vi "Play Preview.vi"() -> ()   [LabVIEW 2013]
doc: "This example VI demonstrates how to acquire and display the preview image from a Phantom Camera using the Vision Research Phantom Series LabVIEW Driver. Also demonstrated is the creation of an image histogram."
uses:
  _Type Defs/PhInt Color.ctl
  _Type Defs/PhInt PhProcessImage Selectors.ctl
  _Type Defs/PhInt REDUCE16TO8PARAMS.ctl
  _Type Defs/PHCon IMRANGE.ctl
  _Type Defs/PhFile InfName.ctl
  _Type Defs/PhFile PRANGE.ctl
  VRI.lvlib
panel:
  in  "REDUCE16TO8PARAMS":T1={"fGain16_8"=1.0}
  in  "procID":T2=1 items=["IMG_PROC_REDUCE16TO8"=1]
  out "Preview":picture
  in  "stop":bool
  in  "Color":T3
  out "pAvgB":u32
  out "pAvgG":u32
  out "pAvgR":u32
  out "Histogram":u32[](graph)
  out "Error Out":errorcluster
  in  "Camera Number":u32
  in  "error in (no error)":errorcluster
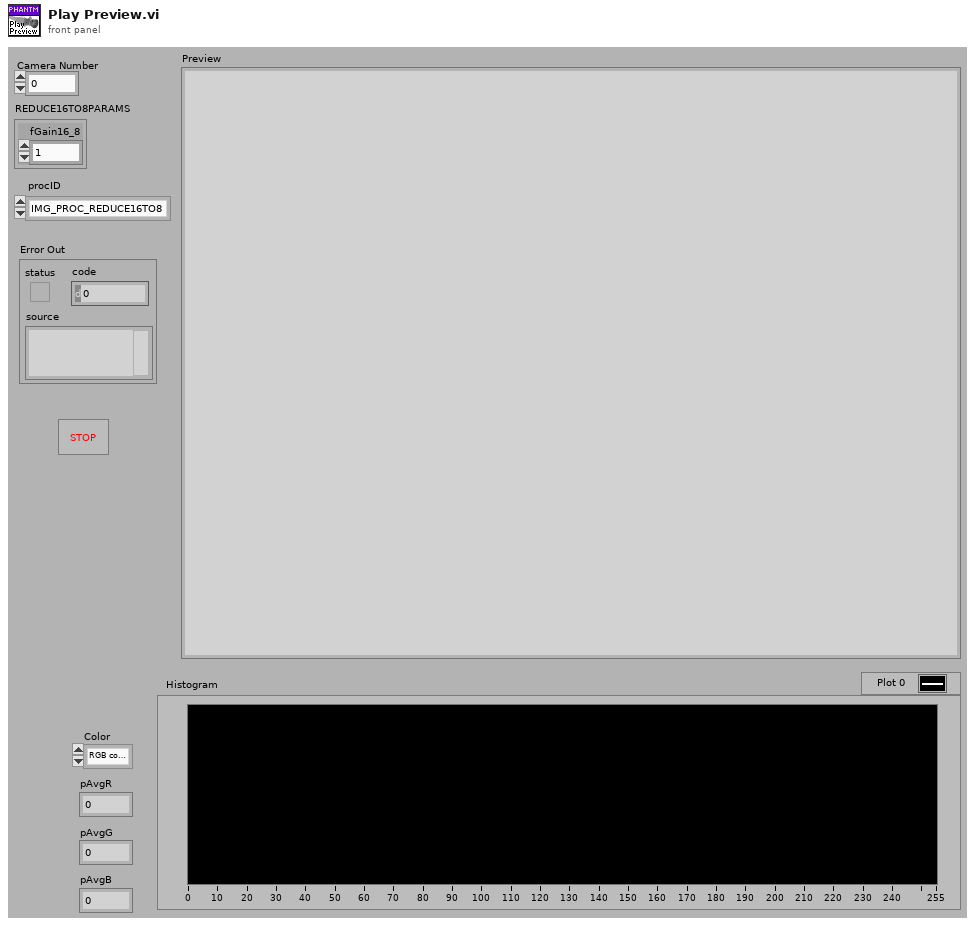
[diagram p1: front panel]
types:
  T1 = typedef "VRI.lvlib/PhInt REDUCE16TO8PARAMS.ctl" = cluster{"fGain16_8":dbl}
  T2 = typedef "VRI.lvlib/PhInt PhProcessImage Selectors.ctl" = u16
  T3 = typedef "VRI.lvlib/PhInt Color.ctl" = enum32{"RGB converted to gray", "RED", "GREEN", "BLUE"}
  T4 = typedef "VRI.lvlib/PhFile PRANGE.ctl" = cluster{"First":u32, "Count":u32}
  T5 = typedef "VRI.lvlib/PhFile InfName.ctl" = u32
  T6 = typedef "VRI.lvlib/PHCon IMRANGE.ctl" = cluster{"First":i32, "Cnt":u32}
  T7 = typedef "VRI.lvlib/PhInt IH.ctl" = cluster{"biSize":u32, "biWidth":i32, "biHeight":i32, "biPlanes":u16, "biBitCount":u16, "biCompresssion":u32, "biSizeImage":u32, "biXPelsPerMeter":i32, "biYPelsPerMeter":i32, "biClrUsed":u32, "biClrImportant":u32, "BlackLevel":i32, "WhiteLevel":i32}
  T8 = typedef "VRI.lvlib/BITMAPINFOHEADER.ctl" = cluster{"biSize":u32, "biWidth":i32, "biHeight":i32, "biPlanes":u16, "biBitCount":u16, "biCompression":u32, "biSizeImage":u32, "biXPelsPerMeter":i32, "biYPelsPerMeter":i32, "biClrUsed":u32, "biClrImportant":u32}
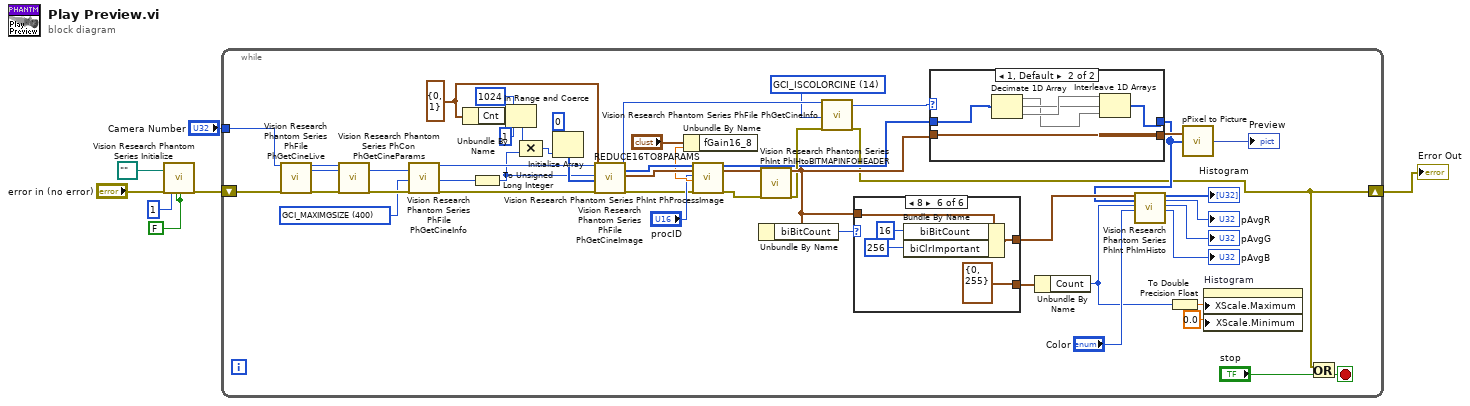
[diagram p0: block diagram]
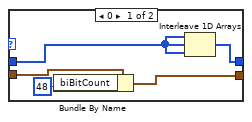
[diagram p2: hidden frame]
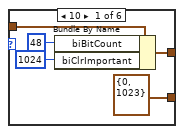
[diagram p3: hidden frame]
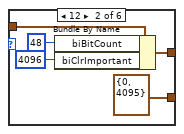
[diagram p4: hidden frame]
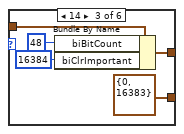
[diagram p5: hidden frame]
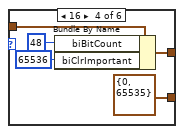
[diagram p6: hidden frame]
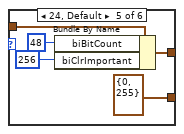
[diagram p7: hidden frame]
diagram:
  w4 = FALSE ("ID Query (T: Check)")
  n1 = call "Vision Research Phantom Series Initialize.vi"("Storage Path (\"\")"=path "" ("Storage Path (\"\")"), "error in (no error)"="error in (no error)", "CallID"=u32 1, "ID Query (T: Check)"=w4, "Reset (F: Don't Reset)"=w4) -> ("Error Out"=w2:errorcluster)  [unwired: 14 out]
  n2 = while {
    tunnel: "Camera Number" -> [w25]
    shift-right: [w8] -> w1
    shift-left: w2 -> [w21]
    stop <- w9 stop-if-true
    w10 = T5 14 items=["GCI_CFA"=0, "GCI_FRAMERATE"=1, "GCI_EXPOSURE"=2, "GCI_AUTOEXPOSURE"=3, "GCI_REALBPP"=4, "GCI_CAMERASERIAL"=5, "GCI_HEADSERIAL0"=6, "GCI_HEADSERIAL1"=7, "GCI_HEADSERIAL2"=8, "GCI_HEADSERIAL3"=9, "GCI_TRIGTIMESEC"=10, "GCI_TRIGTIMEFR"=11, "GCI_ISFILECINE"=12, "GCI_IS16BPPCINE"=13, "GCI_ISCOLORCINE"=14, "GCI_ISMULTIHEADCINE"=15, "GCI_EXPOSURENS"=16, "GCI_EDREXPOSURENS"=17, "GCI_FRAMEDELAYNS"=19, "GCI_FROMFILETYPE"=20, "GCI_COMPRESSION"=21, "GCI_CAMERAVERSION"=22, "GCI_ROTATE"=23, "GCI_IMWIDTH"=24, "GCI_IMHEIGHT"=25, "GCI_IMWIDTHACQ"=26, "GCI_IMHEIGHTACQ"=27, "GCI_POSTTRIGGER"=28, "GCI_IMAGECOUNT"=29, "GCI_TOTALIMAGECOUNT"=30, "GCI_TRIGFRAME"=31, "GCI_AUTOEXPLEVEL"=32, "GCI_AUTOEXPTOP"=33, "GCI_AUTOEXPLEFT"=34, "GCI_AUTOEXPBOTTOM"=35, "GCI_AUTOEXPRIGHT"=36, "GCI_RECORDINGTIMEZONE"=37, "GCI_FIRSTIMAGENO"=38, "GCI_FIRSTMOVIEIMAGE"=39, "GCI_CINENAME"=40, "GCI_FRPSTEPS"=100, "GCI_FRP1X"=101, "GCI_FRP1Y"=102, "GCI_FRP2X"=103, "GCI_FRP2Y"=104, "GCI_FRP3X"=105, "GCI_FRP3Y"=106, "GCI_FRP4X"=107, "GCI_FRP4Y"=108, "GCI_WRITEERR"=109, "GCI_LENSDESCRIPTION"=110, "GCI_LENSAPERATURE"=111, "GCI_LENSFOCALLENGTH"=112, "GCI_WB"=200, "GCI_WBVIEW"=201, "GCI_BRIGHT"=202, "GCI_CONTRAST"=203, "GCI_GAMMA"=204, "GCI_GAMMAR"=223, "GCI_GAMMAB"=224, "GCI_SATURATION"=205, "GCI_HUE"=206, "GCI_FLIPH"=207, "GCI_FLIPV"=208, "GCI_FILTERCODE"=209, "GCI_IMFILTER"=210, "GCI_INTALGO"=211, "GCI_PEDESTALR"=212, "GCI_PEDESTALG"=213, "GCI_PEDESTALB"=214, "GCI_FLARE"=225, "GCI_CHROMA"=226, "GCI_TONE"=227, "GCI_ENABLEMATRICES"=228, "GCI_USERMATRIX"=229, "GCI_RESAMPLEACTIVE"=215, "GCI_RESAMPLEWIDTH"=216, "GCI_RESAMPLEHEIGHT"=217, "GCI_CROPACTIVE"=218, "GCI_CROPRECTANGLE"=219, "GCI_OFFSET16_8"=220, "GCI_GAIN16_8"=221, "GCI_DEMOSAICINGFUNCPTR"=222, "GCI_VFLIPVIEWACTIVE"=300, "GCI_MAXIMGSIZE"=400, "GCI_FRPIMGNOARRAY"=450, "GCI_FRPRATEARRAY"=451, "GCI_FRPSHAPEARRAY"=452, "GCI_TRIGTC"=470, "GCI_TRIGTCU"=471, "GCI_PBRATE"=472, "GCI_TCRATE"=473, "GCI_SAVERANGE"=500, "GCI_SAVEFILENAME"=501, "GCI_SAVEFILETYPE"=502, "GCI_SAVE16BIT"=503, "GCI_SAVEPACKED"=504, "GCI_SAVEXML"=505, "GCI_SAVESTAMPTIME"=506, "GCI_SAVEAVIFRAMERATE"=520, "GCI_SAVEAVICOMPRESSORLIST"=521, "GCI_SAVEAVICOMPRESSORINDEX"=522, "GCI_SAVEDPXLSB"=530, "GCI_SAVEDPXTO10BPS"=531, "GCI_SAVEDPXDATAPACKING"=532, "GCI_SAVEDPX10BITLOG"=533, "GCI_SAVEDPXEXPORTLOGLUT"=534, "GCI_SAVEDPX10BITLOGREFWHITE"=535, "GCI_SAVEDPX10BITLOGREFBLACK"=536, "GCI_SAVEDPX10BITLOGGAMMA"=537, "GCI_SAVEDPX10BITLOGFILMGAMMA"=538, "GCI_SAVEQTPLAYBACKRATE"=550, "GCI_SAVECCIQUALITY"=560, "GCI_UNCALIBRATEDIMAGE"=600, "GCI_NOPROCESSING"=601, "GCI_BADPIXELREPAIR"=602] ("InfName")
    w22 = T5 400 items=["GCI_CFA"=0, "GCI_FRAMERATE"=1, "GCI_EXPOSURE"=2, "GCI_AUTOEXPOSURE"=3, "GCI_REALBPP"=4, "GCI_CAMERASERIAL"=5, "GCI_HEADSERIAL0"=6, "GCI_HEADSERIAL1"=7, "GCI_HEADSERIAL2"=8, "GCI_HEADSERIAL3"=9, "GCI_TRIGTIMESEC"=10, "GCI_TRIGTIMEFR"=11, "GCI_ISFILECINE"=12, "GCI_IS16BPPCINE"=13, "GCI_ISCOLORCINE"=14, "GCI_ISMULTIHEADCINE"=15, "GCI_EXPOSURENS"=16, "GCI_EDREXPOSURENS"=17, "GCI_FRAMEDELAYNS"=19, "GCI_FROMFILETYPE"=20, "GCI_COMPRESSION"=21, "GCI_CAMERAVERSION"=22, "GCI_ROTATE"=23, "GCI_IMWIDTH"=24, "GCI_IMHEIGHT"=25, "GCI_IMWIDTHACQ"=26, "GCI_IMHEIGHTACQ"=27, "GCI_POSTTRIGGER"=28, "GCI_IMAGECOUNT"=29, "GCI_TOTALIMAGECOUNT"=30, "GCI_TRIGFRAME"=31, "GCI_AUTOEXPLEVEL"=32, "GCI_AUTOEXPTOP"=33, "GCI_AUTOEXPLEFT"=34, "GCI_AUTOEXPBOTTOM"=35, "GCI_AUTOEXPRIGHT"=36, "GCI_RECORDINGTIMEZONE"=37, "GCI_FIRSTIMAGENO"=38, "GCI_FIRSTMOVIEIMAGE"=39, "GCI_CINENAME"=40, "GCI_FRPSTEPS"=100, "GCI_FRP1X"=101, "GCI_FRP1Y"=102, "GCI_FRP2X"=103, "GCI_FRP2Y"=104, "GCI_FRP3X"=105, "GCI_FRP3Y"=106, "GCI_FRP4X"=107, "GCI_FRP4Y"=108, "GCI_WRITEERR"=109, "GCI_LENSDESCRIPTION"=110, "GCI_LENSAPERATURE"=111, "GCI_LENSFOCALLENGTH"=112, "GCI_WB"=200, "GCI_WBVIEW"=201, "GCI_BRIGHT"=202, "GCI_CONTRAST"=203, "GCI_GAMMA"=204, "GCI_GAMMAR"=223, "GCI_GAMMAB"=224, "GCI_SATURATION"=205, "GCI_HUE"=206, "GCI_FLIPH"=207, "GCI_FLIPV"=208, "GCI_FILTERCODE"=209, "GCI_IMFILTER"=210, "GCI_INTALGO"=211, "GCI_PEDESTALR"=212, "GCI_PEDESTALG"=213, "GCI_PEDESTALB"=214, "GCI_FLARE"=225, "GCI_CHROMA"=226, "GCI_TONE"=227, "GCI_ENABLEMATRICES"=228, "GCI_USERMATRIX"=229, "GCI_RESAMPLEACTIVE"=215, "GCI_RESAMPLEWIDTH"=216, "GCI_RESAMPLEHEIGHT"=217, "GCI_CROPACTIVE"=218, "GCI_CROPRECTANGLE"=219, "GCI_OFFSET16_8"=220, "GCI_GAIN16_8"=221, "GCI_DEMOSAICINGFUNCPTR"=222, "GCI_VFLIPVIEWACTIVE"=300, "GCI_MAXIMGSIZE"=400, "GCI_FRPIMGNOARRAY"=450, "GCI_FRPRATEARRAY"=451, "GCI_FRPSHAPEARRAY"=452, "GCI_TRIGTC"=470, "GCI_TRIGTCU"=471, "GCI_PBRATE"=472, "GCI_TCRATE"=473, "GCI_SAVERANGE"=500, "GCI_SAVEFILENAME"=501, "GCI_SAVEFILETYPE"=502, "GCI_SAVE16BIT"=503, "GCI_SAVEPACKED"=504, "GCI_SAVEXML"=505, "GCI_SAVESTAMPTIME"=506, "GCI_SAVEAVIFRAMERATE"=520, "GCI_SAVEAVICOMPRESSORLIST"=521, "GCI_SAVEAVICOMPRESSORINDEX"=522, "GCI_SAVEDPXLSB"=530, "GCI_SAVEDPXTO10BPS"=531, "GCI_SAVEDPXDATAPACKING"=532, "GCI_SAVEDPX10BITLOG"=533, "GCI_SAVEDPXEXPORTLOGLUT"=534, "GCI_SAVEDPX10BITLOGREFWHITE"=535, "GCI_SAVEDPX10BITLOGREFBLACK"=536, "GCI_SAVEDPX10BITLOGGAMMA"=537, "GCI_SAVEDPX10BITLOGFILMGAMMA"=538, "GCI_SAVEQTPLAYBACKRATE"=550, "GCI_SAVECCIQUALITY"=560, "GCI_UNCALIBRATEDIMAGE"=600, "GCI_NOPROCESSING"=601, "GCI_BADPIXELREPAIR"=602] ("InfName")
    w26 = T6 {"First"=0, "Cnt"=1} ("pRng")
    n3 = call "Vision Research Phantom Series PhFile PhGetCineLive.vi"("CN (in)"=w25, "Error In (no error)"=w21) -> ("CN (out)"=w32:u32, "pCH (out)"=w46:u32, "Error Out"=w34:errorcluster)  [unwired: 15 in]
    n4 = call "Vision Research Phantom Series PhCon PhGetCineParams.vi"("CN in"=w32, "Error In (no error)"=w34) -> ("Error Out"=w33:errorcluster)  [unwired: 1 in, 16 out]
    n5 = call "Vision Research Phantom Series PhFile PhGetCineInfo.vi"("CH in"=w46, "InfName"=w22, "Error In (no error)"=w33) -> ("CH out"=w44:u32, "pInfVal out"=w14:i32, "Error Out"=w42:errorcluster)  [unwired: 14 in]
    n6 = Unbundle By Name(w26) -> ("Cnt"=w31:u32)
    n7 = To Unsigned Long Integer(number=w14) -> (unsigned 32bit integer=w13:u32)
    n8 = In Range and Coerce(upper limit=u32 1024, x=w31, lower limit=u32 1) -> (coerced(x)=w30:u32)  [unwired: 1 out]
    n9 = Compound Arithmetic op=MULTIPLY(w30, w13) -> (w27:u32)
    n10 = Initialize Array(u16 0 ("element"), w27) -> (w43:u16[])
    n11 = call "Vision Research Phantom Series PhFile PhGetCineImage.vi"("hC [in]"=w44, "pRng [in]"=w26, "bufferByteSize [in]"=w13, "pPixelBuffer [in]"=w43, "Error In (no error)"=w42) -> ("hC [out]"=w20:u32, "pPixelBuffer [out]"=w41:u16[], "IH [out]"=w40:T7, "Error Out"=w37:errorcluster)  [unwired: 11 in]
    n12 = Unbundle By Name("REDUCE16TO8PARAMS") -> ("fGain16_8"=w39:dbl)
    n13 = call "Vision Research Phantom Series PhInt PhProcessImage.vi"("pPixelSrc [in]"=w41, "IH [in]"=w40, "procID"="procID", "pProcParams"=w39, "Error In (no error)"=w37) -> ("pPixelDest [out]"=w11:u8[], "IH [out]"=w35:T7, "Error Out"=w36:errorcluster)  [unwired: 12 in]
    n14 = call "Vision Research Phantom Series PhInt PhIHtoBITMAPINFOHEADER.vi"("IH"=w35, "Error In (no error)"=w36) -> ("BITMAPINFOHEADER"=w17:T8, "Error Out"=w15:errorcluster)  [unwired: 16 in]
    n15 = Unbundle By Name(w17) -> ("biBitCount"=w23:u16)
    n16 = call "Vision Research Phantom Series PhFile PhGetCineInfo.vi"("CH in"=w20, "InfName"=w10, "Error In (no error)"=w15) -> ("pInfVal out"=w19:i32, "Error Out"=w8:errorcluster)  [unwired: 14 in, 1 out]
    n17 = case shown="8" w23 {
      tunnel: [T4 {"First"=0, "Count"=1023} ("PRANGE") T4 {"First"=0, "Count"=4095} ("PRANGE") T4 {"First"=0, "Count"=16383} ("PRANGE") T4 {"First"=0, "Count"=65535} ("PRANGE") T4 {"First"=0, "Count"=255} ("PRANGE") T4 {"First"=0, "Count"=255} ("PRANGE")] -> w24
      tunnel: w17 -> [w70 w75 w80 w85 w90 w96]
      tunnel: [w69 w74 w79 w84 w89 w94] -> w18
      frame 10 {
        n18 = Bundle By Name(cluster=w70, "biBitCount"=u16 48, "biClrImportant"=u32 1024) -> (w69:T8)
      }
      frame 12 {
        n19 = Bundle By Name(cluster=w75, "biBitCount"=u16 48, "biClrImportant"=u32 4096) -> (w74:T8)
      }
      frame 14 {
        n20 = Bundle By Name(cluster=w80, "biBitCount"=u16 48, "biClrImportant"=u32 16384) -> (w79:T8)
      }
      frame 16 {
        n21 = Bundle By Name(cluster=w85, "biBitCount"=u16 48, "biClrImportant"=u32 65536) -> (w84:T8)
      }
      frame 24, Default {
        n22 = Bundle By Name(cluster=w90, "biBitCount"=u16 48, "biClrImportant"=u32 256) -> (w89:T8)
      }
      frame 8 {
        n23 = Bundle By Name(cluster=w96, "biBitCount"=u16 16, "biClrImportant"=u32 256) -> (w94:T8)
      }
    }
    n24 = case shown="1, Default" w19 {
      tunnel: [w59 w63] -> w12
      tunnel: w17 -> [w62 w68]
      tunnel: [w61 w68] -> w16
      tunnel: w11 -> [w58 w64]
      frame 0 {
        n25 = Bundle By Name(cluster=w62, "biBitCount"=u16 48) -> (w61:T8)
        n26 = Interleave 1D Arrays(w58, w58, w58) -> (w59:u8[])
      }
      frame 1, Default {
        n27 = Decimate 1D Array(w64) -> (w65:u8[], w66:u8[], w67:u8[])
        n28 = Interleave 1D Arrays(w67, w66, w65) -> (w63:u8[])
      }
    }
    n29 = Unbundle By Name(w24) -> ("Count"=w49:u32)
    n30 = call "Vision Research Phantom Series PhInt PhImHisto.vi"("pBMIH"=w18, "pPixel In"=w12, "HistoSize"=w49, "Color"="Color") -> ("pHisto"=→"Histogram":u32[], "pAvgR"=→"pAvgR":u32, "pAvgG"=→"pAvgG":u32, "pAvgB"=→"pAvgB":u32)  [unwired: 1 in, 11 out]
    n31 = To Double Precision Float(number=w49) -> (double precision float=w56:dbl)
    n32 = call "pPixel to Picture.vi"("pPixel"=w12, "BITMAPINFOHEADER"=w16) -> ("Preview"=→"Preview":picture)  [unwired: 1 in]
    n33 = property on="Histogram" class="WFGraph (strict)"("XScale.Maximum"=w56, "XScale.Minimum"=0.0 ("X Scale.Range:Minimum")) -> ()  [unwired: 2 in, 2 out]
    n34 = Or(x=w8, y="stop") -> (x .or. y?=w9:bool)
  }
  "Error Out" <- w1
